vi "Dispense FN - ON (SubVI).vi"(0 "Signals IN":T3, 1 "Values IN":T2 {"Drain Time (s)" format="%.2f"; "Drain Rate (g/sec)" format="%.2f"}, 2 "Settings":T1={"ON Settings"={"Enable Dynamic Setpoint?"=TRUE, "Enable Dynamic Dispense Time?"=TRUE, "Enable Drain Rate Functions"=TRUE, "Dispense Sample Time (s)"=0.5, "Dispense Slope Ave"=0, "ON Timeout (sec)"=600.0, "1st Setpoint (% of Target)"=0.0, "2nd Setpoint (% of Target)"=0.0, "3rd Setpoint (% of Target)"=0.0, "Measure Dispense Delay (sec)"=0.0, "Settle Slope Sample Time (s)"=0.0}, "OFF Settings"={"Drain Sample Time (s)"=0.5, "Drain Rate Ave Size"=5, "Drain Rate Limits (± g/sec)"=10.0, "Level Slope Range (± g/sec)"=0.25, "OFF Timeout (sec)"=0.0, "Near SP Slope Level (± g/sec)"=0.01, "Near Setpoint Threshold (%)"=95.0}, "Overshoot Settings"={"Time Limit (s)"=60.0, "Container MAX (g)"=1500.0, "Max FILL Slope (+/- g/sec)"=10.0, "% Overshot to Enable (>)"=0.25}, "FILL Timeout (s)"=300.0, "Full Settle Time (s)"=20.0, "Pre-Hydrate \nSpray Time (s)"=10.0, "Pre-Hydrate \nWait Time (s)"=30.0}, 3 "Main Concentration Setpoint (%)":dbl, 4 "Measured Mass (g)":dbl, 5 "State Change?":bool, 7 "Main Case Change?":bool) -> (14 "Signals OUT":T3, 15 "Values OUT":T2 {"Drain Time (s)" format="%.2f"; "Drain Rate (g/sec)" format="%.2f"}, 19 "OFF Signal":bool)   [LabVIEW 2012]
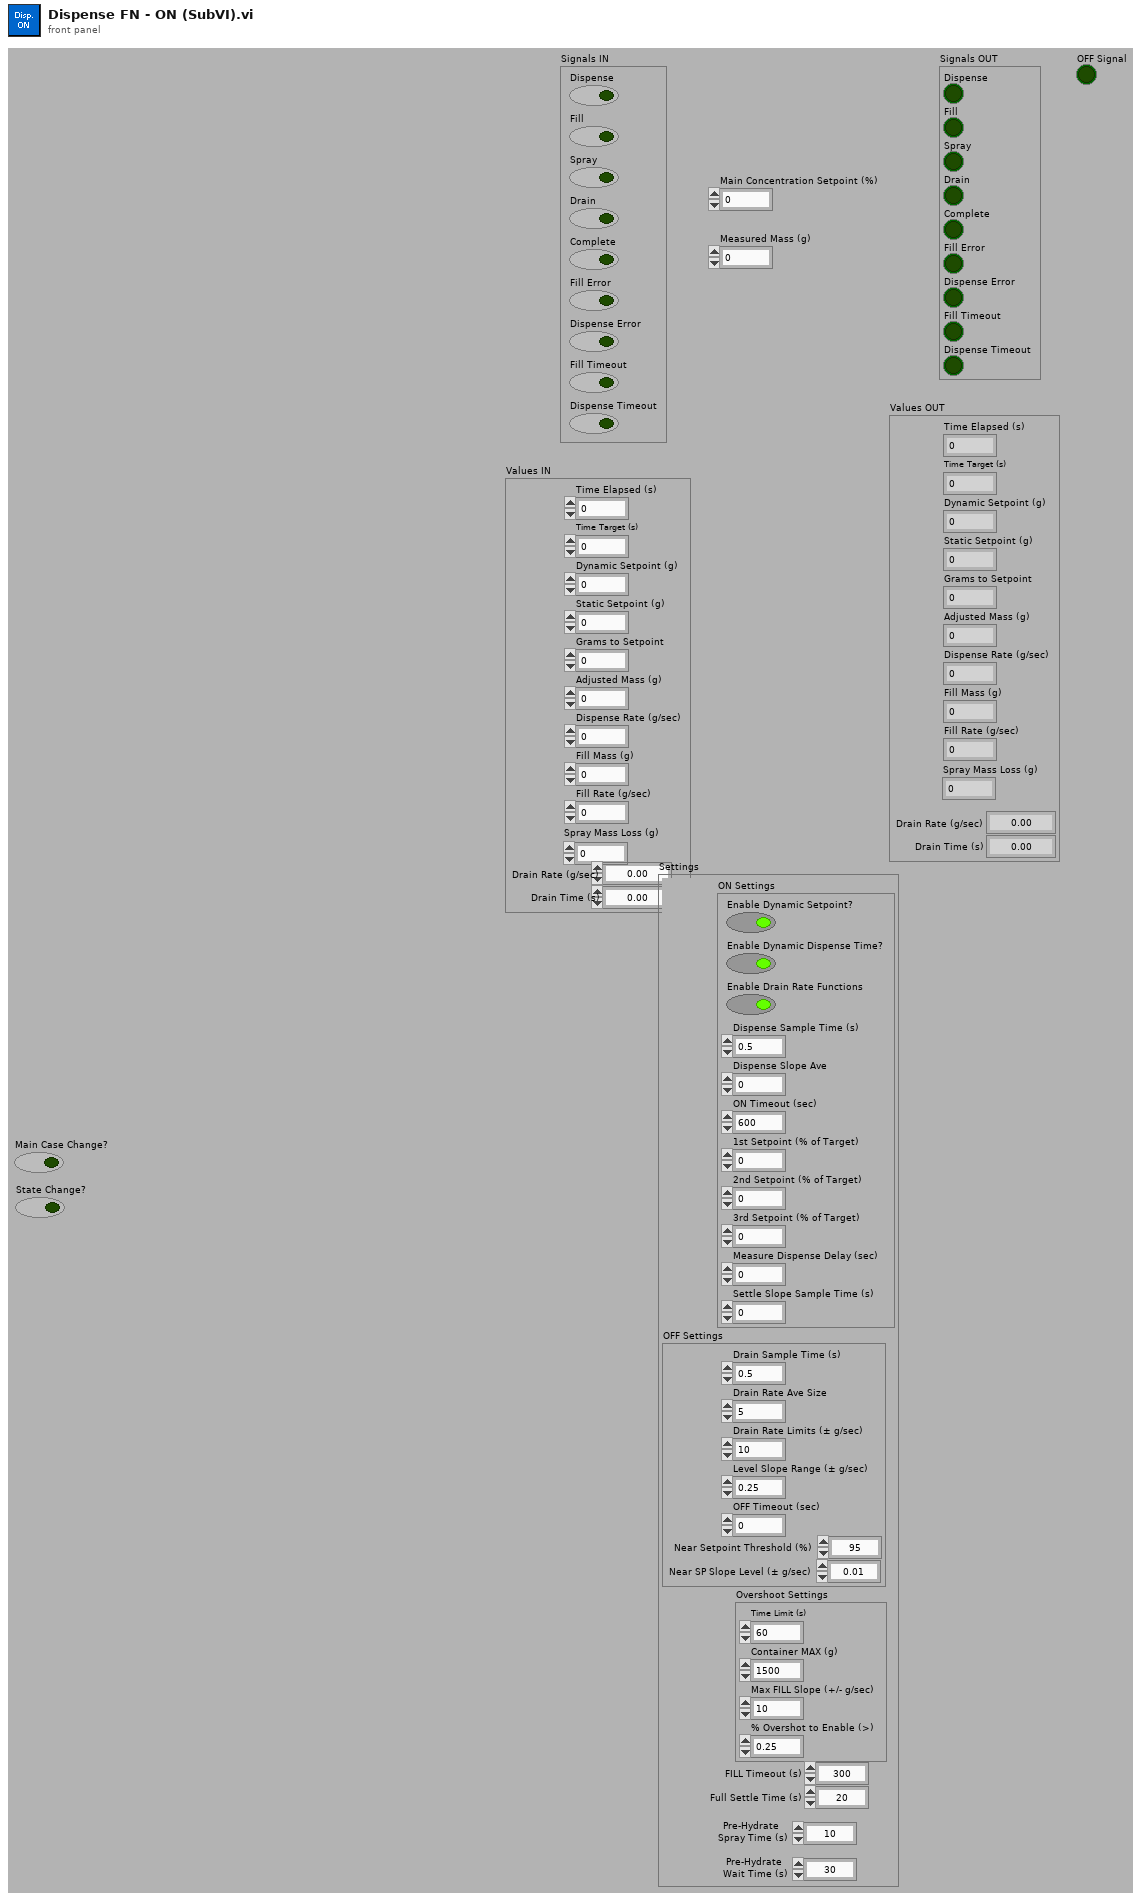
[diagram p1: front panel]
types:
  T1 = cluster{"ON Settings":cluster{"Enable Dynamic Setpoint?":bool, "Enable Dynamic Dispense Time?":bool, "Enable Drain Rate Functions":bool, "Dispense Sample Time (s)":dbl, "Dispense Slope Ave":i32, "ON Timeout (sec)":dbl, "1st Setpoint (% of Target)":dbl, "2nd Setpoint (% of Target)":dbl, "3rd Setpoint (% of Target)":dbl, "Measure Dispense Delay (sec)":dbl, "Settle Slope Sample Time (s)":dbl}, "OFF Settings":cluster{"Drain Sample Time (s)":dbl, "Drain Rate Ave Size":i32, "Drain Rate Limits (± g/sec)":dbl, "Level Slope Range (± g/sec)":dbl, "OFF Timeout (sec)":dbl, "Near SP Slope Level (± g/sec)":dbl, "Near Setpoint Threshold (%)":dbl}, "Overshoot Settings":cluster{"Time Limit (s)":dbl, "Container MAX (g)":dbl, "Max FILL Slope (+/- g/sec)":dbl, "% Overshot to Enable (>)":dbl}, "FILL Timeout (s)":dbl, "Full Settle Time (s)":dbl, "Pre-Hydrate \nSpray Time (s)":dbl, "Pre-Hydrate \nWait Time (s)":dbl}
  T2 = cluster{"Time Elapsed (s)":dbl, "Time Target (s)":dbl, "Dynamic Setpoint (g)":dbl, "Static Setpoint (g)":dbl, "Grams to Setpoint":dbl, "Adjusted Mass (g)":dbl, "Dispense Rate (g/sec)":dbl, "Fill Mass (g)":dbl, "Fill Rate (g/sec)":dbl, "Spray Mass Loss (g)":dbl, "Drain Rate (g/sec)":dbl, "Drain Time (s)":dbl}
  T3 = cluster{"Dispense":bool, "Fill":bool, "Spray":bool, "Drain":bool, "Complete":bool, "Fill Error":bool, "Dispense Error":bool, "Fill Timeout":bool, "Dispense Timeout":bool}
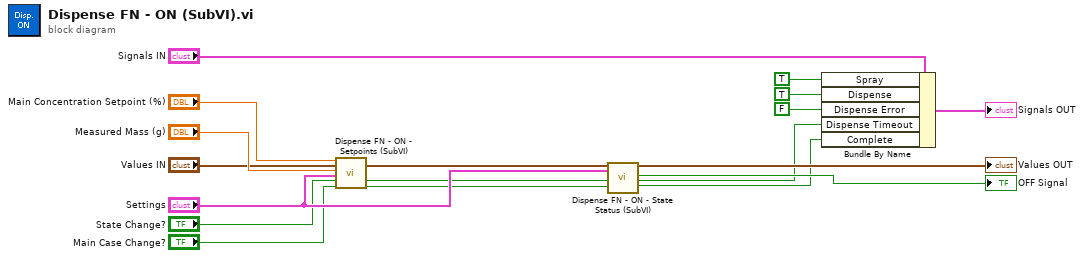
[diagram p0: block diagram]
diagram:
  n1 = call "Dispense FN - ON - Setpoints (SubVI).vi"("Main Concentration Setpoint (%)"="Main Concentration Setpoint (%)", "Values IN"="Values IN", "Measured Mass (g)"="Measured Mass (g)", "Settings"="Settings", "State Change?"="State Change?", "Main Case Change?"="Main Case Change?") -> ("Values OUT"=w10:T2, "Dynamic SP Valid?"=w4:bool, "Enable Dispense Measure?"=w9:bool)  [unwired: 11 out]
  n2 = call "Dispense FN - ON - State Status (SubVI).vi"("Values IN"=w10, "Settings"="Settings", "Dynamic SP Valid?"=w4, "Enable Dispense Measure?"=w9) -> ("Values OUT"=→"Values OUT":T2, "OFF Signal"=→"OFF Signal":bool, "Dispense Timeout?"=w8:bool, "Complete"=w7:bool)  [unwired: 6 in, 6 out]
  n3 = Bundle By Name(cluster="Signals IN", "Spray"=TRUE, "Dispense"=TRUE, "Dispense Error"=FALSE, "Dispense Timeout"=w8, "Complete"=w7) -> (→"Signals OUT":T3)
